vi "ziListNodesJSON.vi"(0 "Handle In":T2 {"Handle" format="0x%08x"; "Conn" format="0x%08x"}, 5 "Path (\"\")":string, 9 "Flags (None)":T3, 11 "Error In":errorcluster) -> (4 "Handle Out":T2 {"Handle" format="0x%08x"; "Conn" format="0x%08x"}, 6 "Doc":T1(array[cluster]), 15 "Error Out":errorcluster)   [LabVIEW 2009, in "Zurich Instruments LabOne.lvlib"]
doc: "Returns <b> nodes documentation </b> found at the specified path. The path may contain wild cards so that the rertuned nodes do not necessarily have to have the same parents."
uses:
  <instrlib>/Zurich Instruments LabOne/Zurich Instruments LabOne.lvlib
  <instrlib>/Zurich Instruments LabOne/Public/ziTypeHandle.ctl
  <vilib>/regexp/Match Regular Expression.xnode
  <instrlib>/Zurich Instruments LabOne/Private/ziLV32.dll
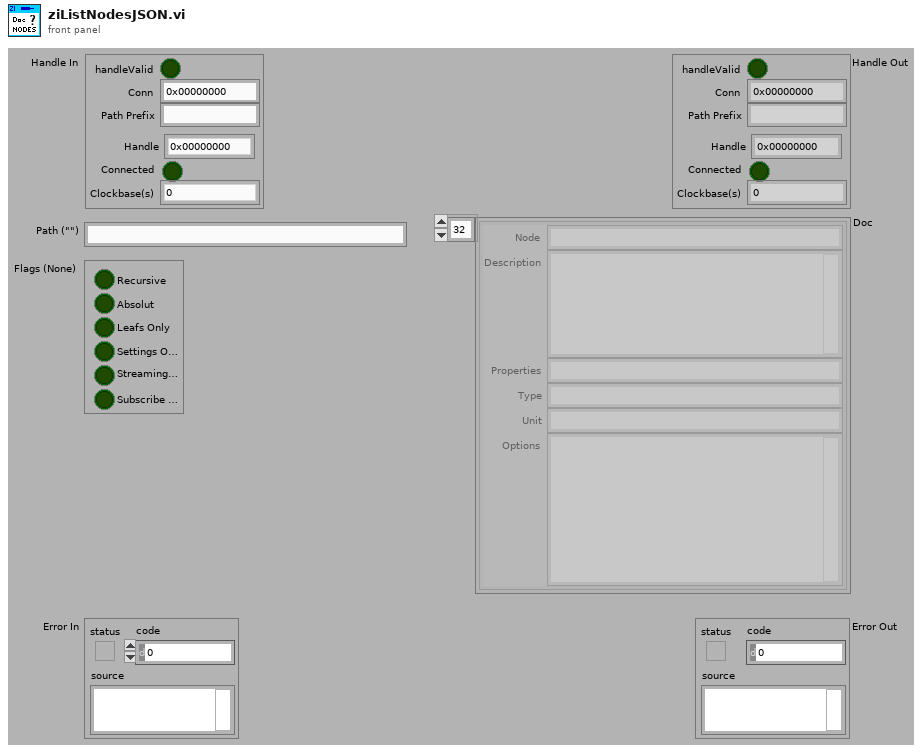
[diagram p1: front panel]
types:
  T1 = cluster{"Node":string, "Description":string, "Properties":string, "Type":string, "Unit":string, "Options":string}[]
  T2 = typedef "Zurich Instruments LabOne.lvlib/ziTypeHandle.ctl" = cluster{"handleValid":bool, "Conn":u64, "Path Prefix":string, "Handle":u64, "Connected":bool, "Clockbase(s)":dbl}
  T3 = cluster{"Recursive":bool, "Absolut":bool, "Leafs Only":bool, "Settings Only":bool, "Streaming Only":bool, "Subscribe Only":bool}
  T4 = cluster{"Node":string, "Description":string, "Properties":string, "Type":string, "Unit":string, "Options":string}
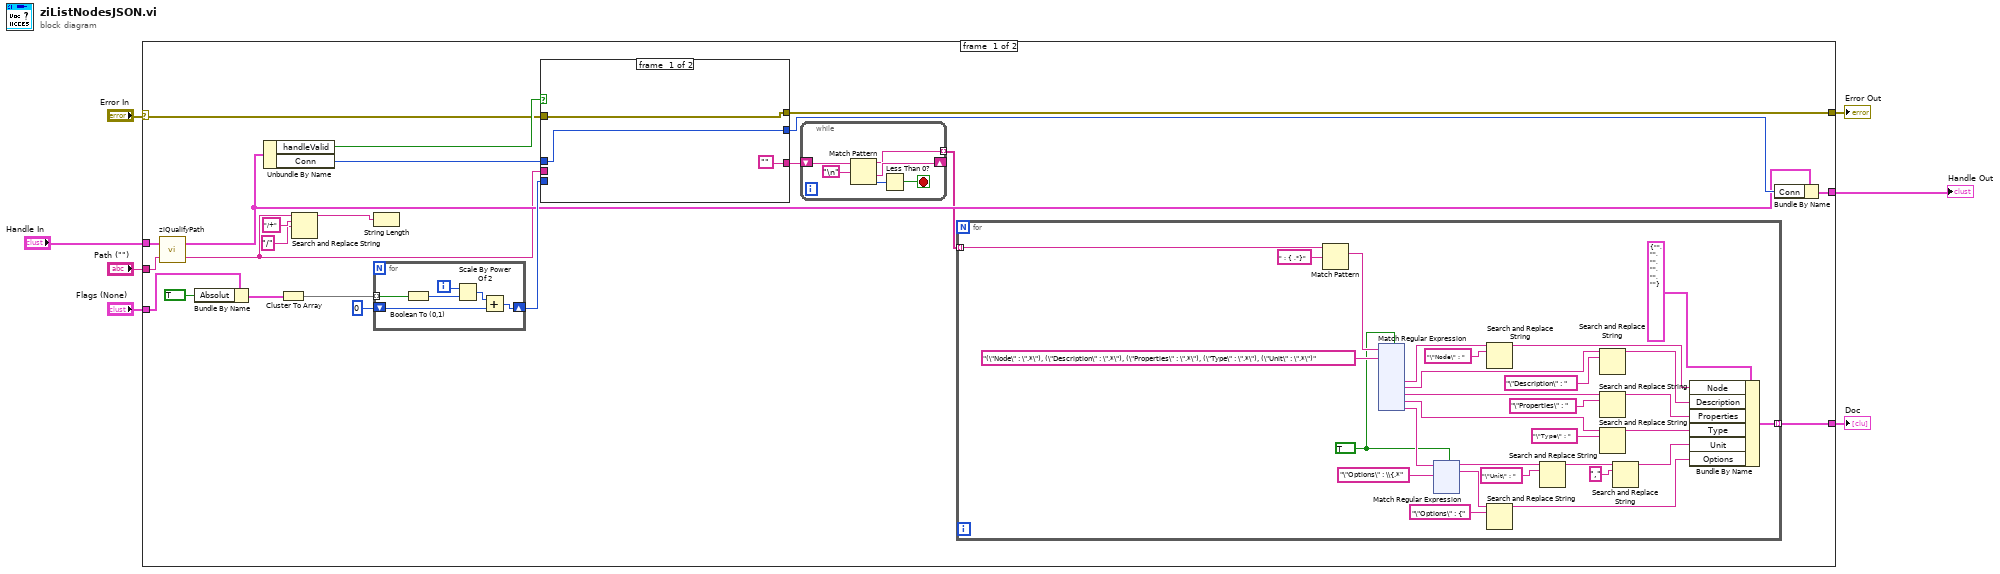
[diagram p0: block diagram]
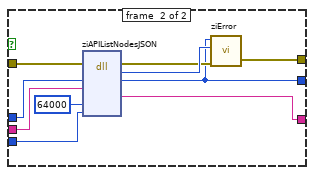
[diagram p2: hidden frame]
diagram:
  n1 = case shown="No Error" "Error In" {
    selector: "Error In" -> [w11 w305]
    tunnel: [w29 w305] -> w7
    tunnel: [w22 w304] -> w6
    tunnel: "Path (\"\")" -> [w21 _]
    tunnel: "Handle In" -> [w20 w304]
    tunnel: "Flags (None)" -> [w17 _]
    tunnel: [w8 _] -> w1
    frame #0 {
      n2 = call <instrlib>:"ziQualifyPath.vi"("Path In"=w21, "Handle In"=w20) -> ("Path Out"=w12:string, "Handle Out"=w19:T2)
      n3 = Bundle By Name(cluster=w17, "Absolut"=TRUE) -> (w16:T3)
      n4 = Unbundle By Name(w19) -> ("handleValid"=w28:bool, "Conn"=w27:u64)
      n5 = Cluster To Array(cluster=w16) -> (array=w25:bool[])
      n6 = Search and Replace String(input string=w12, search string="/+" ("replace string (\"\")"), replace string="/" ("replace string (\"\")")) -> (result string=w13:string)  [unwired: 2 in, 6 out]
      n7 = String Length(string=w13) -> ()  [unwired: 1 out]
      n8 = for {
        tunnel: w25 -> [w290] mode=indexing
        shift-right: [w286] -> w23
        shift-left: 0 -> [w287]
        i -> [w285]
        n9 = Boolean To (0,1)(Boolean=w290) -> (0, 1=w289:i16)
        n10 = Scale By Power Of 2(n=w285, x=w289) -> (x*2^n=w288:i16)
        n11 = Add(x=w288, y=w287) -> (x+y=w286:i32)
      }
      n12 = case shown="True" w28 {
        tunnel: ["" w302] -> w9
        tunnel: w11 -> [w292 w300]
        tunnel: w27 -> [w291 w301]
        tunnel: [w291 w294] -> w26
        tunnel: [w292 w295] -> w29
        tunnel: w12 -> [_ w298]
        tunnel: w23 -> [_ w303]
        frame #0 {
        }
        frame #1 {
          n13 = dll-call lib="C:/Program Files (x86)/National Instruments/LabVIEW 2009/instr.lib/Zurich Instruments LabOne/Private/ziLV*.*" fn="ziAPIListNodesJSON"(error in=w300, "Conn"=w301, "Path"=w298, "MaxLen"=64000, "Flags"=w303) -> (error out=w296:errorcluster, "return type"=w297:u32, "Conn"=w294:u64, "Nodes"=w302:string)  [unwired: 5 in, 2 out]
          n14 = call <instrlib>:"ziError.vi"("Conn"=w294, "ziErrorCode"=w297, "Error In"=w296) -> ("Error Out"=w295:errorcluster)  [unwired: 2 in, 1 out]
        }
      }
      n15 = while {
        shift-right: [w282] -> _
        shift-left: w9 -> [w284]
        tunnel: [w280] -> w10 mode=indexing
        stop <- w279 stop-if-true
        n16 = Match Pattern(string=w284, regular expression="\n") -> (before substring=w280:string, after substring=w282:string, offset past match=w281:i32)  [unwired: 1 in, 1 out]
        n17 = Less Than 0?(x=w281) -> (x < 0?=w279:bool)
      }
      n18 = for {
        tunnel: w10 -> [w58] mode=indexing
        tunnel: [w30] -> w8 mode=indexing
        w52 = TRUE ("multiline? (F)")
        n19 = Match Pattern(string=w58, regular expression=" : { .*}") -> (match substring=w56:string)  [unwired: 1 in, 3 out]
        n20 = xnode "Match Regular Expression"("input string"=w56, "regular expression"="(\"Node\" : \".*\"), (\"Description\" : \".*\"), (\"Properties\" : \".*\"), (\"Type\" : \".*\"), (\"Unit\" : \".*\")", "multiline? (F)"=w52) -> ("submatch 1"=w51:string, "submatch 2"=w48:string, "submatch 3"=w47:string, "submatch 4"=w34:string, "submatch 5"=w53:string)  [unwired: 3 in, 5 out]
        n21 = xnode "Match Regular Expression"("input string"=w53, "regular expression"="\"Options\" : \\{.*", "multiline? (F)"=w52) -> ("before match"=w40:string, "whole match"=w36:string)  [unwired: 3 in, 3 out]
        n22 = Search and Replace String(input string=w51, search string="\"Node\" : ") -> (result string=w50:string)  [unwired: 6 in, 3 out]
        n23 = Search and Replace String(input string=w36, search string="\"Options\" : {" ("substring (\"\")")) -> (result string=w35:string)  [unwired: 6 in, 3 out]
        n24 = Search and Replace String(input string=w40, search string="\"Unit\" : ") -> (result string=w32:string)  [unwired: 6 in, 3 out]
        n25 = Search and Replace String(input string=w48, search string="\"Description\" : ") -> (result string=w49:string)  [unwired: 6 in, 3 out]
        n26 = Search and Replace String(input string=w47, search string="\"Properties\" : ") -> (result string=w46:string)  [unwired: 6 in, 3 out]
        n27 = Search and Replace String(input string=w34, search string="\"Type\" : ") -> (result string=w41:string)  [unwired: 6 in, 3 out]
        n28 = Search and Replace String(input string=w32, search string=",") -> (result string=w31:string)  [unwired: 6 in, 3 out]
        n29 = Bundle By Name(cluster=T4 {"Node"="", "Description"="", "Properties"="", "Type"="", "Unit"="", "Options"=""} ("output cluster 2"), "Node"=w50, "Description"=w49, "Properties"=w46, "Type"=w41, "Unit"=w31, "Options"=w35) -> (w30:T4)
      }
      n30 = Bundle By Name(cluster=w19, "Conn"=w26) -> (w22:T2)
    }
    frame #1 {
    }
  }
  "Error Out" <- w7
  "Doc" <- w1
  "Handle Out" <- w6
